vi "BSCAN_DEMO05_Zynq_I2C_STLM75.vi"() -> ()   [LabVIEW 2017]
uses:
  Saldigi_protocol_library.lvlibp/HAL/HAL_version_typedef.ctl
  Saldigi_protocol_library.lvlibp
panel:
  out "dt":dbl(graph)=0.03743209999993269
  in  "I2C typedef in":T2={"SDA padded"=[], "CLK padded"=[], "String array"=[], "Slave addr 7bit"=73, "clocked bits"=0, "output rate"=0.0, "SDA channel name"="chain0/xc7z020_clg400/IO_P15", "CLK channel name"="chain0/xc7z020_clg400/IO_P16", "SDA-IN channel name"="", "Version"=enum."BSCAN V2", "Parameter string"=""} {"Slave addr 7bit" format="%07b"}
  out "I2C ACK OK":bool=TRUE
  out "error out":errorcluster
  out "Celcius":dbl=32.625 format="%#.6g"
  in  "stop":bool
  # "69ms"
  # "saldigi.fi protocol library"
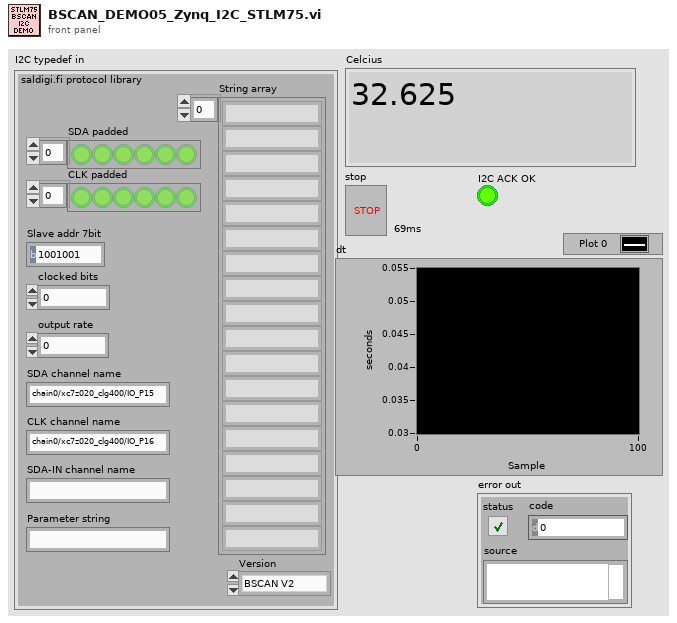
[diagram p1: front panel]
types:
  T1 = typedef "Saldigi_protocol_library.lvlibp/HAL_version_typedef.ctl" = enum16{"DAQmx V1", "DAQmx V2", "FTn232H", "BSCAN V1", "DAQmx V1.1", "DAQmx V2.1", "J-LINK BSCAN", "BSCAN V2"}
  T2 = cluster{"SDA padded":bool[], "CLK padded":bool[], "String array":string[], "Slave addr 7bit":u8, "clocked bits":i32, "output rate":dbl, "SDA channel name":string, "CLK channel name":string, "SDA-IN channel name":string, "Version":T1, "Parameter string":string}
  T3 = typedef "Saldigi_protocol_library.lvlibp/I2C_typedef.ctl" = cluster{"SDA padded":bool[], "CLK padded":bool[], "String array":string[], "Slave addr 7bit":u8, "clocked bits":i32, "output rate":dbl, "SDA channel name":string, "CLK channel name":string, "SDA-IN channel name":string, "Version":T1, "Parameter string":string}
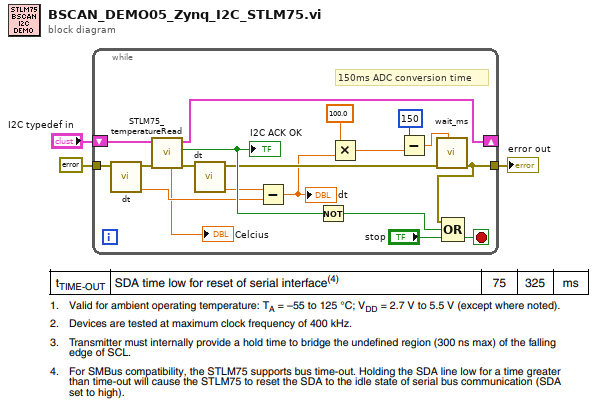
[diagram p0: block diagram]
diagram:
  n1 = while {
    tunnel: errorcluster {"status"=FALSE, "code"=0, "source"=""} ("error in") -> [w15]
    tunnel: [w18] -> w1
    shift-right: [w19] -> _
    shift-left: "I2C typedef in" -> [w21]
    stop <- w20 stop-if-true
    # "150ms ADC conversion time"
    n2 = call "dt.vi"("error in"=w15) -> ("relative seconds"=w10:dbl, "error out"=w14:errorcluster)  [unwired: 9 in]
    n3 = call "STLM75_temperatureRead.vi"("error in"=w14, "I2C typedef in"=w21) -> ("error out"=w13:errorcluster, "I2C ACK OK"=w17:bool, "I2C typedef out"=w19:T3, "Celcius out"=→"Celcius":dbl)  [unwired: 6 in]
    "I2C ACK OK" <- w17
    n4 = call "dt.vi"("error in"=w13) -> ("relative seconds"=w11:dbl, "error out"=w12:errorcluster)  [unwired: 9 in]
    n5 = Subtract(x=w11, y=w10) -> (x-y=w7:dbl)
    "dt" <- w7
    n6 = Not(x=w17) -> (.not. x?=w16:bool)
    n7 = Multiply(x=100.0, y=w7) -> (x*y=w5:dbl)
    n8 = Subtract(x=u32 150 ("milliseconds to wait"), y=w5) -> (x-y=w6:dbl)
    n9 = call "wait_ms.vi"("milliseconds to wait"=w6, "error in"=w12) -> ("error out"=w18:errorcluster)  [unwired: 9 in]
    n10 = Compound Arithmetic op=OR(w18, w16, "stop") -> (w20:bool)
  }
  "error out" <- w1
